vi "rqcBob Get Bitfile path.vi"(6 "bitfile version":string, 8 "error in":errorcluster, 9 "Device":string, 10 "Resource Name":string) -> (0 "error out":errorcluster, 1 "rqcBob Bitfile path":path, 2 "Resource Name out":string, 3 "Device out":string)   [LabVIEW 2019, in "rqcBob.lvclass"]
uses:
  rqcBob.lvclass
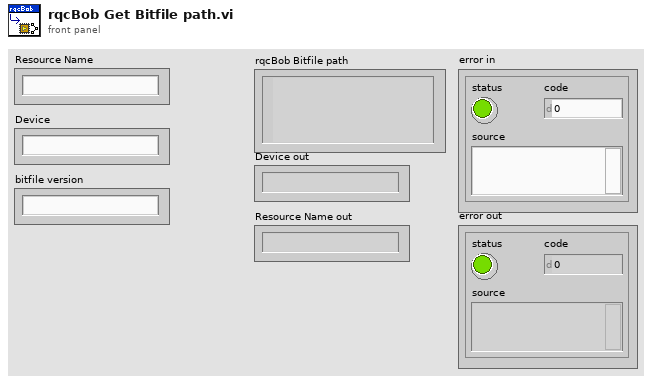
[diagram p1: front panel]
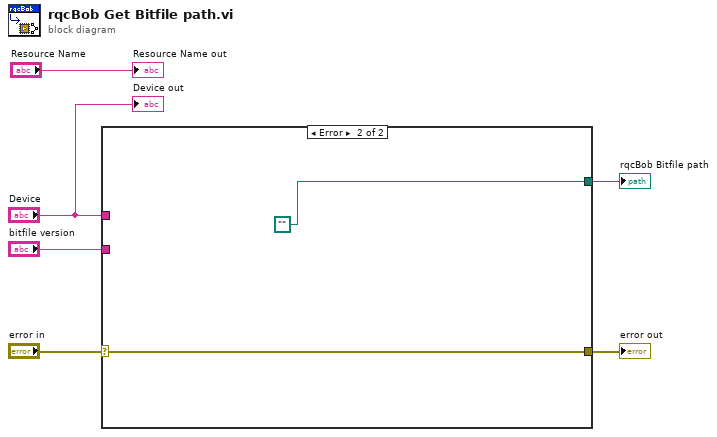
[diagram p0: block diagram]
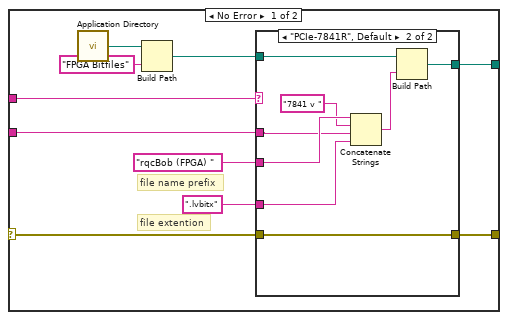
[diagram p2: hidden frame]
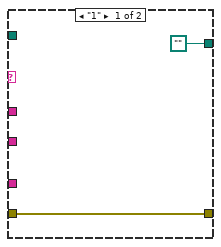
[diagram p3: hidden frame]
diagram:
  n1 = case shown="Error" "error in" {
    selector: "error in" -> [w14 w28]
    tunnel: [w13 w28] -> w5
    tunnel: "Device" -> [w16 _]
    tunnel: [w15 path ""] -> w2
    tunnel: "bitfile version" -> [w7 _]
    frame No Error {
      # "file extention"
      # "file name prefix"
      n2 = call <vilib>:"Application Directory.vi"() -> ("Application Directory"=w12:path)
      n3 = Build Path(base path=w12, name or relative path="FPGA Bitfiles") -> (appended path=w10:path)
      n4 = case shown="\"PCIe-7841R\", Default" w16 {
        tunnel: [path "" w19] -> w15
        tunnel: w14 -> [w17 w26]
        tunnel: [w17 w26] -> w13
        tunnel: w10 -> [_ w21]
        tunnel: "rqcBob (FPGA) " ("name or relative path") -> [_ w25]
        tunnel: ".lvbitx" ("name or relative path") -> [_ w22]
        tunnel: w7 -> [_ w23]
        frame "1" {
        }
        frame "PCIe-7841R", Default {
          n5 = Concatenate Strings(w25, "7841 v " ("name or relative path"), w23, w22) -> (w20:string)
          n6 = Build Path(base path=w21, name or relative path=w20) -> (appended path=w19:path)
        }
      }
    }
    frame Error {
    }
  }
  "error out" <- w5
  "rqcBob Bitfile path" <- w2
  "Device out" <- "Device"
  "Resource Name out" <- "Resource Name"
